vi "Gas Rack MAIN (RT).vi"() -> ()   [LabVIEW 2013]
uses:
  TypeDef/Controller Names.ctl
  TypeDef/Command Cluster.ctl
  TypeDef/DataCluster.ctl
  TCP/PC/Event Mode.ctl
  CAN Communication/CAN Mode.ctl
  TCP/RT/RTsend PCrecv CMD.ctl
  RT subVIs/Controls/Stream RT FIFO Mode.ctl
  TypeDef/TCP Cluster.ctl
  TypeDef/Stability Cluster.ctl
  <vilib>/FPGAPlugInAG/sbRIO-9626/niLvFpga_Open_sbRIO-9626.vi
  <vilib>/rvi/interface/common/dynamic/niFpgaDynamicAddResources.vi
  <vilib>/rvi/interface/common/niFpgaWaitOnOcc.vi
  <vilib>/Utility/error.llb/Error Cluster From Error Code.vi
  <vilib>/rvi/errors/niLvFpgaAdjustHostInterfaceError.vi
  <vilib>/FPGAPlugInAG/Dynamic/niLvFpga_Reset_Dynamic.vi
  <vilib>/FPGAPlugInAG/Dynamic/niLvFpga_Run_Dynamic.vi
  <vilib>/rvi/interface/nirviOpenFPGA/nirviOpenFPGA.xnode
  FPGA Bitfiles/Portable Gas Rack.lvbitx
  FPGA/Portable Gas Rack Main (FPGA).vi
  <vilib>/rvi/interface/nirviReadWriteControl/nirviReadWriteControl.xnode
  <vilib>/rvi/interface/nirviMethod/nirviMethod.xnode
  <vilib>/NI_Real-Time Target Support.lvlib
  <vilib>/rvi/interface/Simulation/niFpgaSimulationCallBeginRW.vi
  <vilib>/ptbypt/NI_PtbyPt.lvlib
  <vilib>/FPGAPlugInAG/Dynamic/niLvFpga_ReadFifo_Dynamic.vi
  <vilib>/rvi/errors/niLvFpgaMergeErrorWithErrorCode.vi
  NiFpgaLv.dll
panel:
  in  "DesiredCluster":T1
  in  "Enable Graphs":bool
  out "time 3":dbl
  out "time 2":dbl
  out "time":dbl
  out "Ave Data Cluster":T2 {"Efficiency (%)" format="%#_6f"; "Speed (RPM)" format="%#.1f"; "Fuel Temp (C)" format="%.1f"; "Controller Current (A)" format="%.2f"; "Controller Voltage (V)" format="%.2f"; "Flow (L/H)" format="%.1f"; "Pressure (kPA)" format="%.1f"; "Pump Current (Arms)" format="%.2f"; "Pump Voltage (V)" format="%#.2f"}
  in  "Tab Control Config":enum32{"PID/slew", "Cal/Hidden"}(tab)
  in  "SaveConfig":bool
  in  "ControlArray":T3(array[cluster])=[{"Name"="Volt_Direct", "PI Far->Close"=[], "FFinfo"={"FF_m"=0.0, "FF_b"=0.0}, "Limits"={"StepSize"=1e-05, "Max"=10.0, "Min"=0.0, "IndMin"=0.0}}, {"Name"="Volt_Flow", "PI Far->Close"=[], "FFinfo"={"FF_m"=0.0, "FF_b"=0.0}, "Limits"={"StepSize"=1e-05, "Max"=10.0, "Min"=0.0, "IndMin"=0.0}}, {"Name"="Volt_Speed", "PI Far->Close"=[], "FFinfo"={"FF_m"=0.0, "FF_b"=0.0}, "Limits"={"StepSize"=1e-05, "Max"=10.0, "Min"=0.0, "IndMin"=0.0}}, {"Name"="Pres_Direct", "PI Far->Close"=[], "FFinfo"={"FF_m"=0.0, "FF_b"=0.0}, "Limits"={"StepSize"=1e-05, "Max"=10.0, "Min"=0.0, "IndMin"=0.0}}, {"Name"="Pres_Flow", "PI Far->Close"=[], "FFinfo"={"FF_m"=0.0, "FF_b"=0.0}, "Limits"={"StepSize"=1e-05, "Max"=10.0, "Min"=0.0, "IndMin"=0.0}}, {"Name"="Pres_Speed", "PI Far->Close"=[], "FFinfo"={"FF_m"=0.0, "FF_b"=0.0}, "Limits"={"StepSize"=1e-05, "Max"=10.0, "Min"=0.0, "IndMin"=0.0}}, {"Name"="CMD_Direct", "PI Far->Close"=[], "FFinfo"={"FF_m"=0.0, "FF_b"=0.0}, "Limits"={"StepSize"=1e-05, "Max"=10.0, "Min"=0.0, "IndMin"=0.0}}, {"Name"="CMD_Flow", "PI Far->Close"=[], "FFinfo"={"FF_m"=0.0, "FF_b"=0.0}, "Limits"={"StepSize"=1e-05, "Max"=10.0, "Min"=0.0, "IndMin"=0.0}}, {"Name"="CMD_Speed", "PI Far->Close"=[], "FFinfo"={"FF_m"=0.0, "FF_b"=0.0}, "Limits"={"StepSize"=1e-05, "Max"=10.0, "Min"=0.0, "IndMin"=0.0}}]
  out "Speed":dbl
  in  "Max Window":dbl=1400.0 format="%.4f"
  in  "Min Window":dbl=300.0 format="%.4f"
  in  "CAN CMD":u16
  out "Speed Loop Time":dbl
  out "Actual Loop Time 2":u32
  in  "Count 2(uS)":u32=35
  out "Actual Loop Time":u32
  in  "Count 1(uS)":u32=100
  in  "Brushed Speed":bool
  in  "Stream Stop":bool
  in  "CommSegs":i32
  out "PrevCalDate":i32
  in  "CmdCluster":T1
  out "PresSig":dbl
  out "VSig":dbl
  in  "VDirect":dbl
  in  "DirectV?":bool
  in  "DirectPres?":bool
  in  "PresDirect":dbl
  in  "PS Enable":bool
  out "Controller Name":T4
  out "Total (%)":dbl
  in  "GraphTab":enum32{"Page 1", "Page 2"}(tab)=enum."Page 2"
  out "WFG1":dbl[][](graph)
  out "WFG2":dbl[][](graph)
  out "WFG3":dbl[][](graph)
  out "WFG6":dbl[][](graph)
  out "WFG5":dbl[][](graph)
  out "WFG4":dbl[][](graph)
  # "Should be 0.1"
  # "CalDate is frozen to 3/8/17"
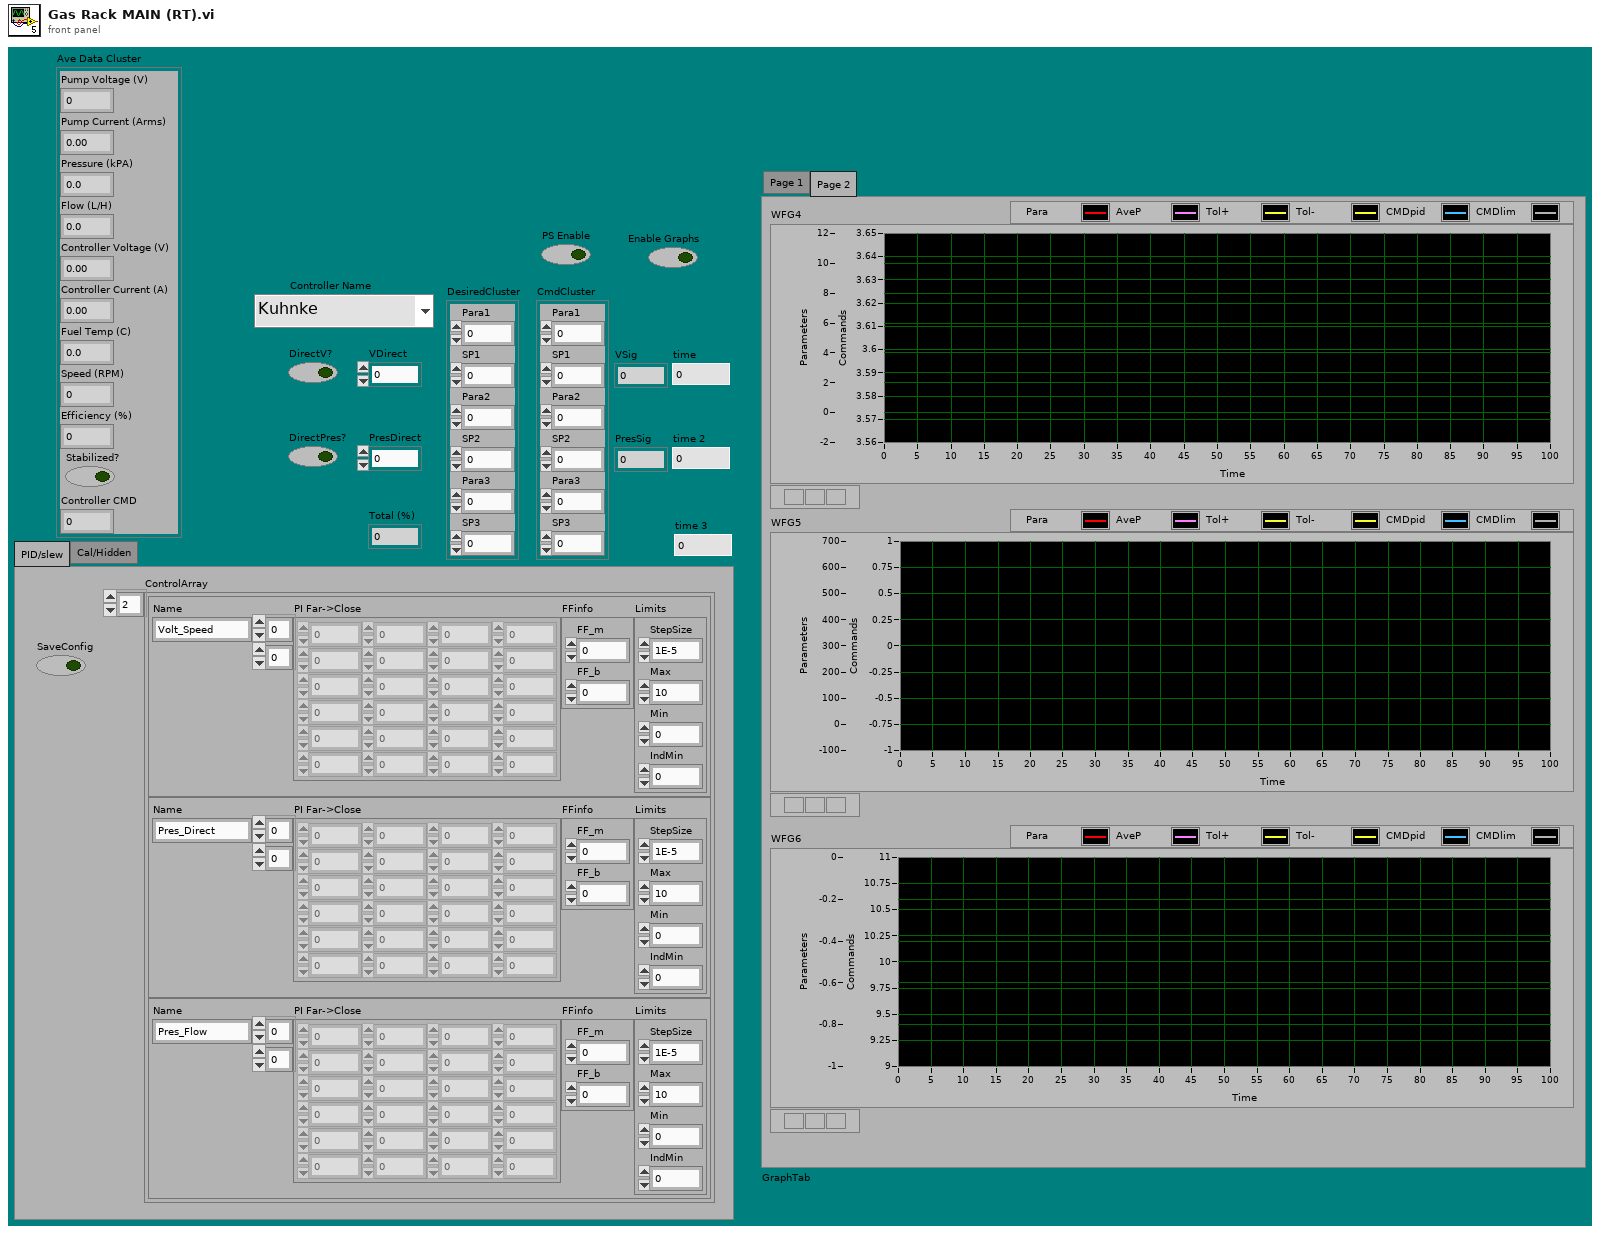
[diagram p1: front panel]
types:
  T1 = typedef "Command Cluster.ctl" = cluster{"Para1":i32, "SP1":dbl, "Para2":i32, "SP2":dbl, "Para3":i32, "SP3":dbl}
  T2 = typedef "DataCluster.ctl" = cluster{"Pump Voltage (V)":dbl, "Pump Current (Arms)":dbl, "Pressure (kPA)":dbl, "Flow (L/H)":dbl, "Controller Voltage (V)":dbl, "Controller Current (A)":dbl, "Fuel Temp (C)":dbl, "Speed (RPM)":dbl, "Efficiency (%)":dbl, "Stabilized?":bool, "Controller CMD":dbl}
  T3 = cluster{"Name":string, "PI Far->Close":dbl[][], "FFinfo":cluster{"FF_m":dbl, "FF_b":dbl}, "Limits":cluster{"StepSize":dbl, "Max":dbl, "Min":dbl, "IndMin":dbl}}[]
  T4 = typedef "Controller Names.ctl" = enum16{"Kuhnke", "McLaren", "Helbako BLDC", "Conti", "Hella E4LMF", "Hella E4LMD", "Hella E4DCG 20mm", "Hella E4DCG 30mm", "Helbako (old)", "TI PWM", "PSA", "Hella Hyundai Gas", "Hella Hyundai Diesel", "8 Comm", "10 Comm", "8 Comm Hella FCA", "10 Comm Hella FCA", "8 Comm Omron", "10 Comm Omron", "8 Comm Nissan", "10 Comm Nissan"}
  T5 = cluster{"Controller Name":T4, "CommSeg":i32, "PWM?":bool, "Frequency":i32, "Low Command":dbl, "High Command":dbl, "Stop Command":dbl, "Command Step":dbl, "Solenoid Stop?":bool, "Controller?":bool, "Name":string, "Indirect Nonzero CMD":dbl}[]
  T6 = cluster{"Controller Name":T4, "CommSeg":i32, "PWM?":bool, "Frequency":i32, "Low Command":dbl, "High Command":dbl, "Stop Command":dbl, "Command Step":dbl, "Solenoid Stop?":bool, "Controller?":bool, "Name":string, "Indirect Nonzero CMD":dbl}
  T7 = cluster{"Name":string, "PI Far->Close":cluster{"Slew":dbl, "Kp":dbl, "Ki":dbl}[], "Limits":cluster{"StepSize":dbl, "Max":dbl, "Min":dbl}, "Cutoffs":cluster{"Middle":dbl, "Close":dbl}, "FFinfo":cluster{"FF_m":dbl, "FF_b":dbl}}[]
  T8 = cluster{"Stability Reads":i32, "Stability1":i32, "Stability2":i32, "Stability3":i32}
  T9 = typedef "RTsend PCrecv CMD.ctl" = enum16{"Data", "Connected?", "CalFileDate"}
  T10 = typedef "CAN Mode.ctl" = enum16{"Init", "Read", "Write", "Close"}
  T11 = typedef "Event Mode.ctl" = enum16{"Init", "Get", "Set", "Destroy"}
  T12 = cluster{"CommandCluster":T1, "Deadhead?":bool, "FPGA Data Rate (sec)":dbl, "FPGA Data Timer":dbl, "PC Data Rate (sec)":dbl, "PC Data Timer":dbl, "InstDataCluster":T2, "Controller":cluster{"Controller Name":T4, "CommSeg":i32, "PWM?":bool, "Frequency":i32, "Low Command":dbl, "High Command":dbl, "Stop Command":dbl, "Command Step":dbl, "Solenoid Stop?":bool, "Controller?":bool, "Name":string, "Indirect Nonzero CMD":dbl}, "PWM Period (ticks)":u32, "Tolerances":dbl[], "Cal Coeffs":dbl[][], "PS Enable":bool, "StabilityCluster":cluster{"Stability Reads":i32, "Stability1":i32, "Stability2":i32, "Stability3":i32}, "AveDataCluster":T2, "CMD Scaler":dbl, "Controller List":cluster{"Controller Name":T4, "CommSeg":i32, "PWM?":bool, "Frequency":i32, "Low Command":dbl, "High Command":dbl, "Stop Command":dbl, "Command Step":dbl, "Solenoid Stop?":bool, "Controller?":bool, "Name":string, "Indirect Nonzero CMD":dbl}[], "VandPLimit":dbl[], "FreezeCmdPID":bool, "DesiredCluster":T1, "Version":u8, "ControlArray":cluster{"Name":string, "PI Far->Close":dbl[][], "FFinfo":cluster{"FF_m":dbl, "FF_b":dbl}, "Limits":cluster{"StepSize":dbl, "Max":dbl, "Min":dbl, "IndMin":dbl}}[], "TolBands":dbl[][], "NeedleValve":bool}
  T13 = typedef "TCP Cluster.ctl" = cluster{"Command":string, "FlattenedData":string}
  T14 = cluster{"CommandCluster":T1, "DesiredCluster":T1}
  T15 = typedef "Stream RT FIFO Mode.ctl" = enum16{"Create", "Write", "Read", "Delete"}
  T16 = typedef "PCsend RTrecv CMD.ctl" = enum16{"ConnSettings", "Connect", "CMD", "Controller", "PSenable", "ReqCalDate", "Tolerances", "Stable Trigger", "Stop", "VPLimits", "NeedleValve", "SpeedWindow", "FreezeCmdPID"}
  T17 = typedef "Stability Cluster.ctl" = cluster{"Voltage Tolerances":dbl, "Pressure Tolerances":dbl, "Flow Tolerances":dbl, "Speed Tolerances":dbl, "Stable Count (sec)":dbl}
  T18 = cluster{"Pump Voltage":fxp<+/-,25,15>, "Pump Current":fxp<+/-,25,15>, "Pressure":fxp<+/-,25,15>, "Flow":fxp<+/-,25,15>, "Controller Voltage":fxp<+/-,25,15>, "Controller Current":fxp<+/-,25,15>, "Temperature":fxp<+/-,25,15>, "Speed":fxp<+/-,25,15>}
  T19 = cluster{"[0]":dbl, "[1]":dbl, "[2]":dbl, "[3]":dbl, "[4]":dbl, "[5]":dbl, "[6]":dbl, "[7]":dbl}
  T20 = typedef "NI_Real-Time Target Support.lvlib/RT CPU Load.ctl" = cluster{"Total (%)":dbl, "Time Critical (%)":dbl, "Timed Structures (%)":dbl, "High (%)":dbl, "Above Normal (%)":dbl, "Normal (%)":dbl, "Background (%)":dbl, "Idle (%)":dbl, "ISR (%)":dbl}
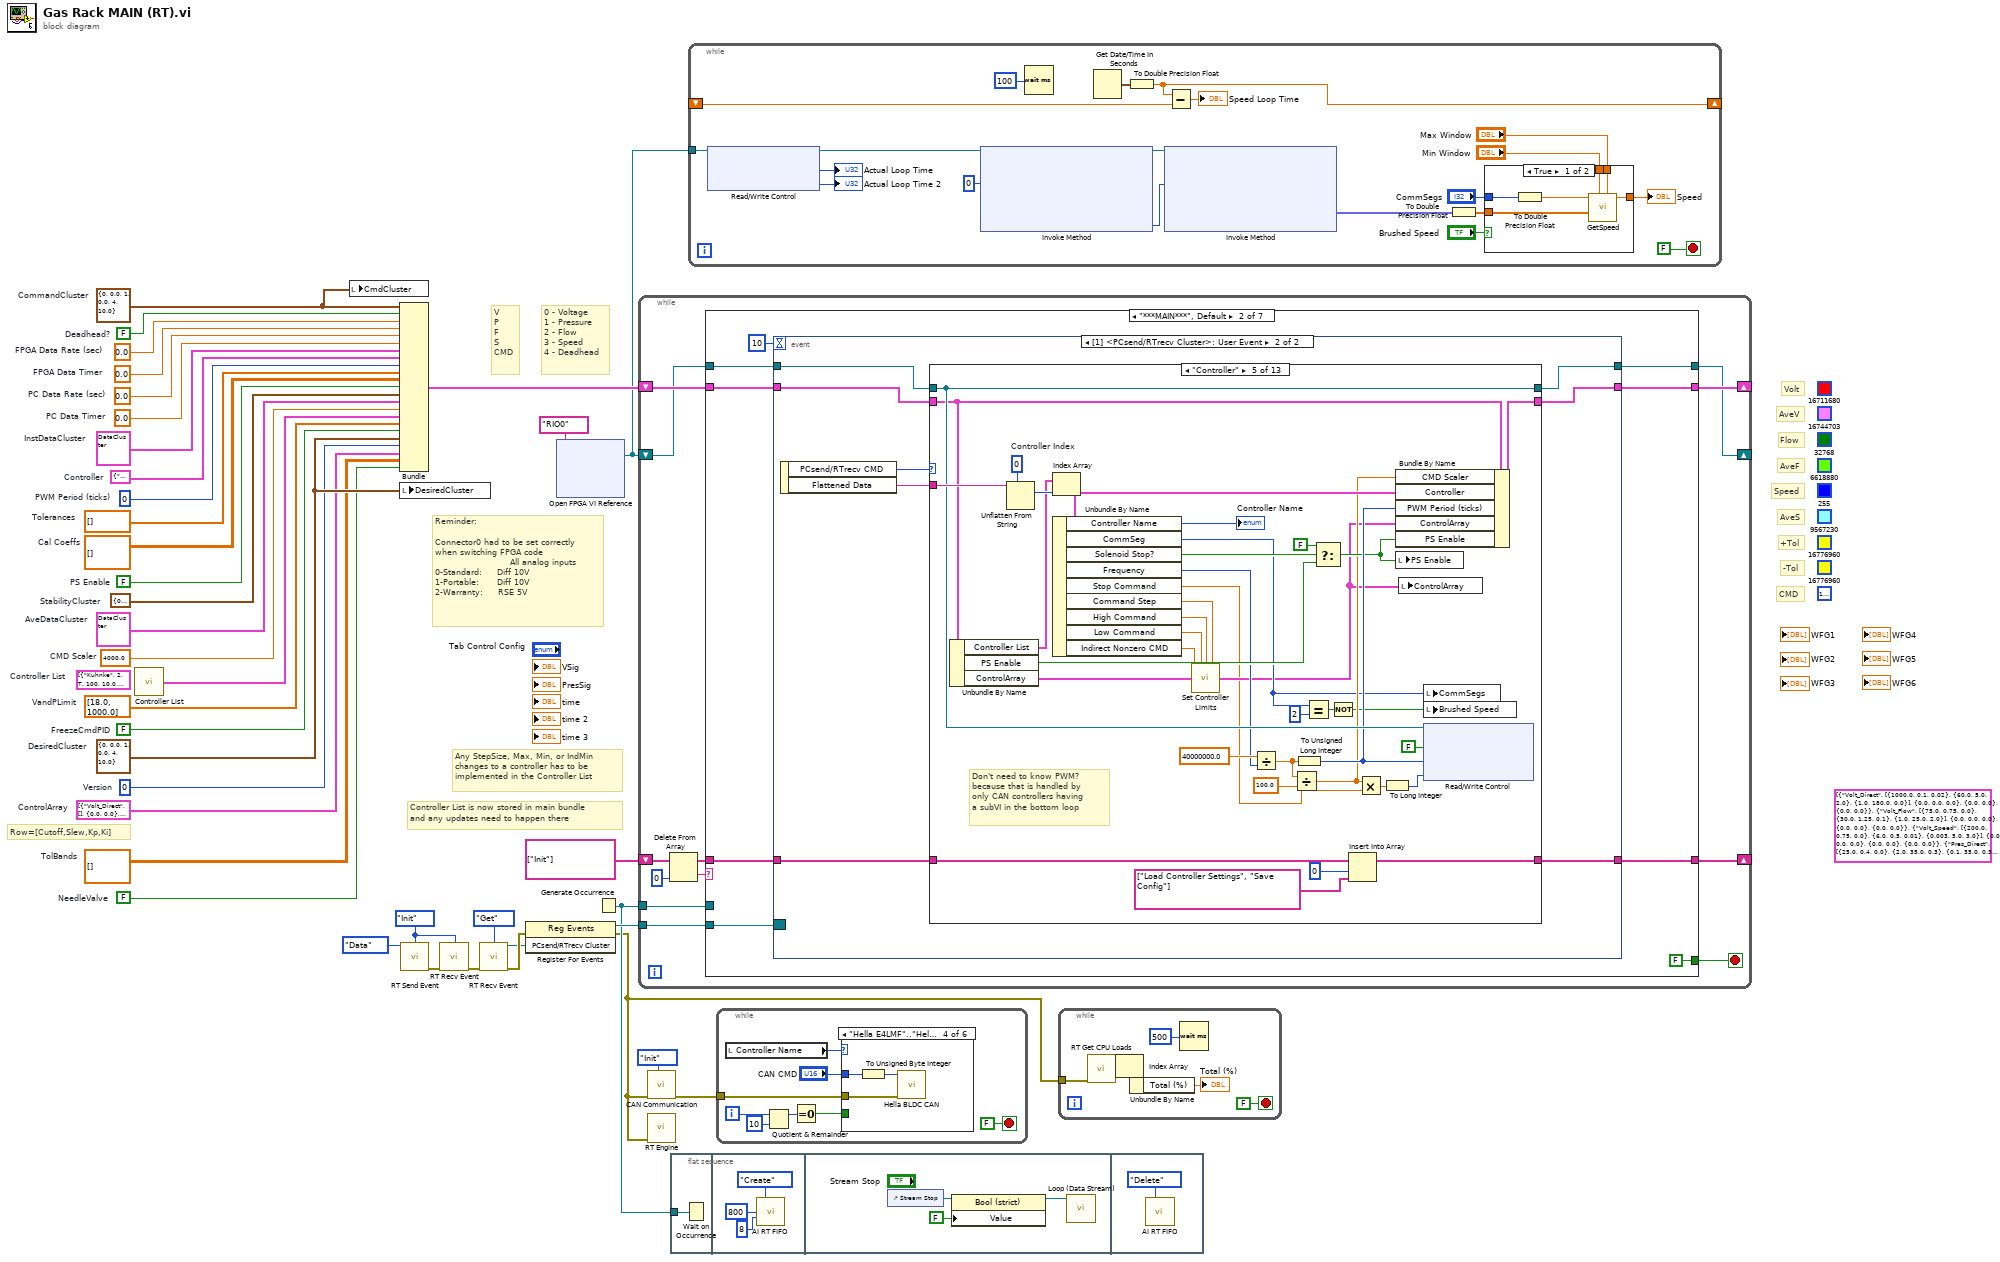
[diagram p0: block diagram]
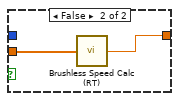
[diagram p2: hidden frame]
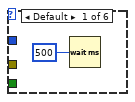
[diagram p3: hidden frame]
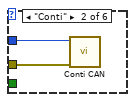
[diagram p4: hidden frame]
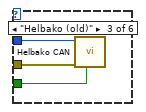
[diagram p5: hidden frame]
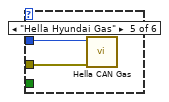
[diagram p6: hidden frame]
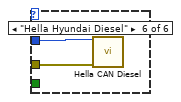
[diagram p7: hidden frame]
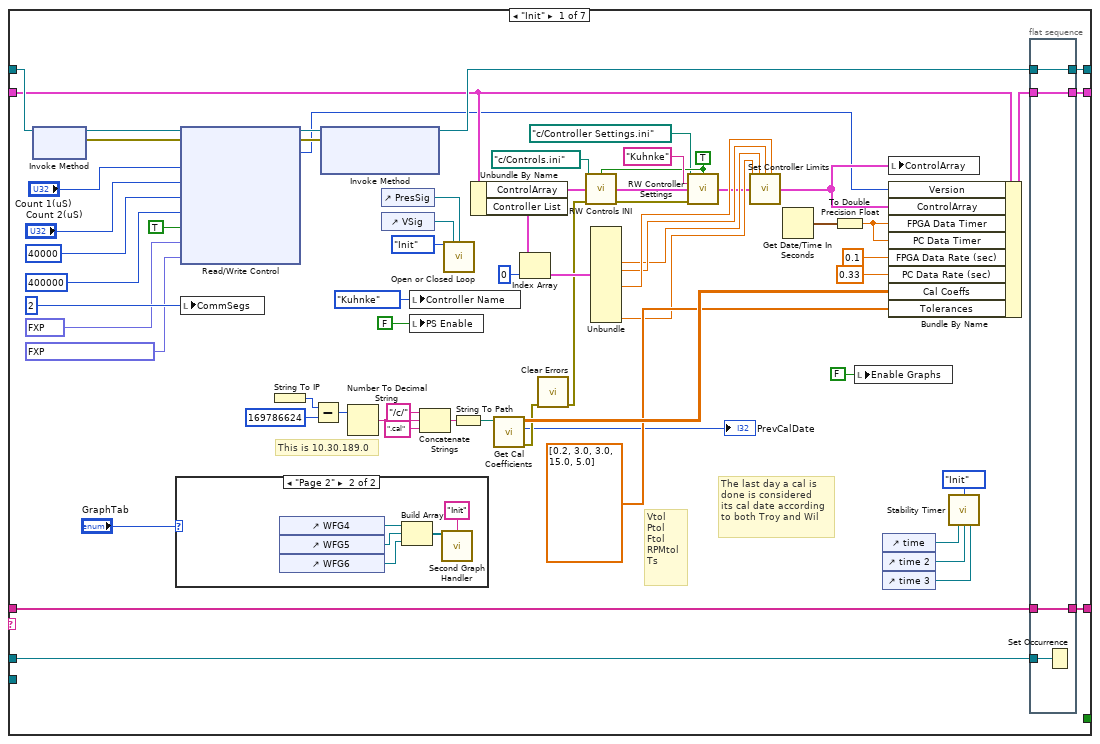
[diagram p8: hidden frame]
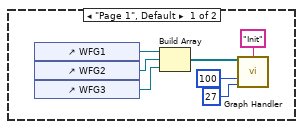
[diagram p9: hidden frame]
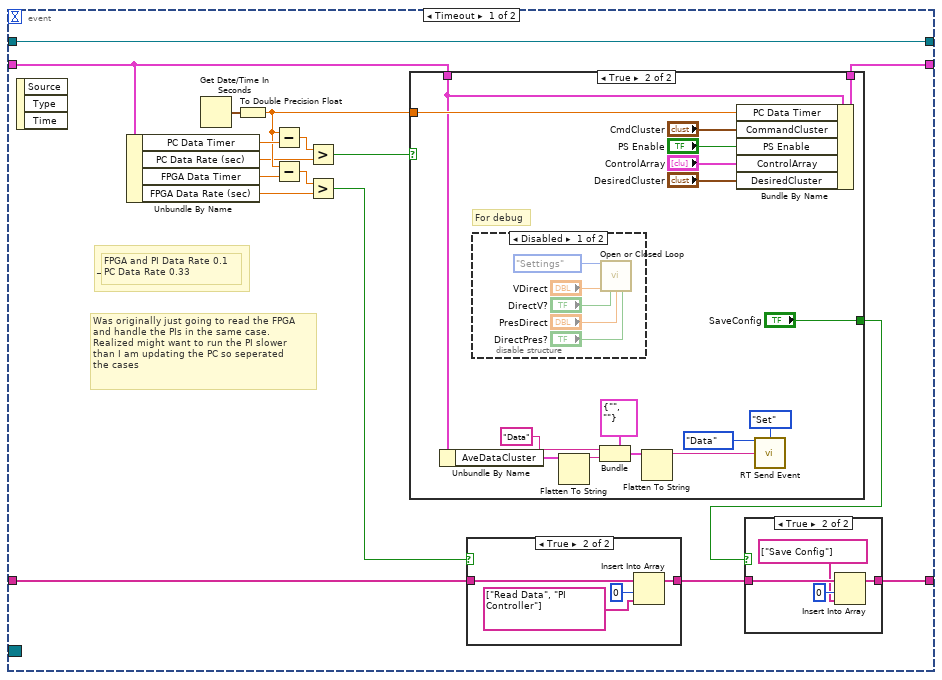
[diagram p10: hidden frame]
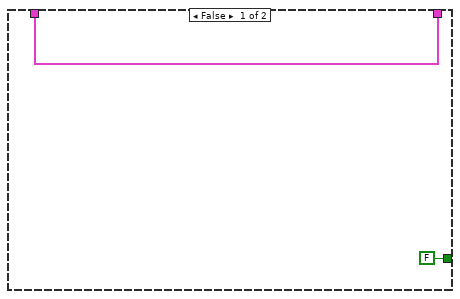
[diagram p13: hidden frame]
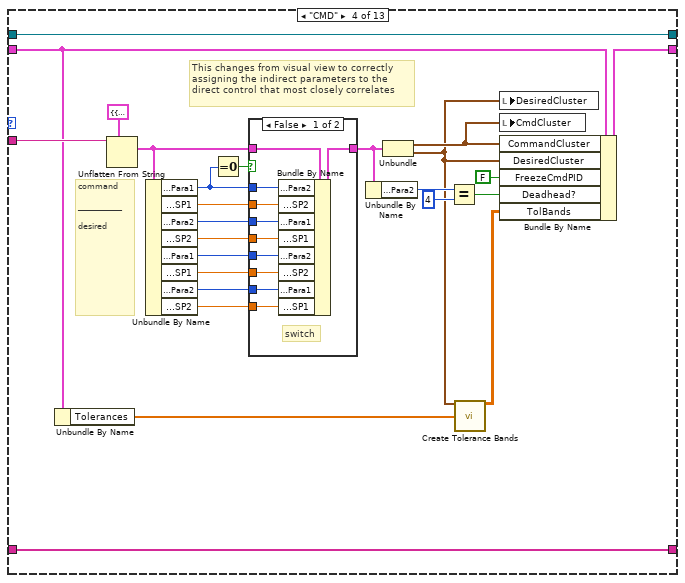
[diagram p18: hidden frame]
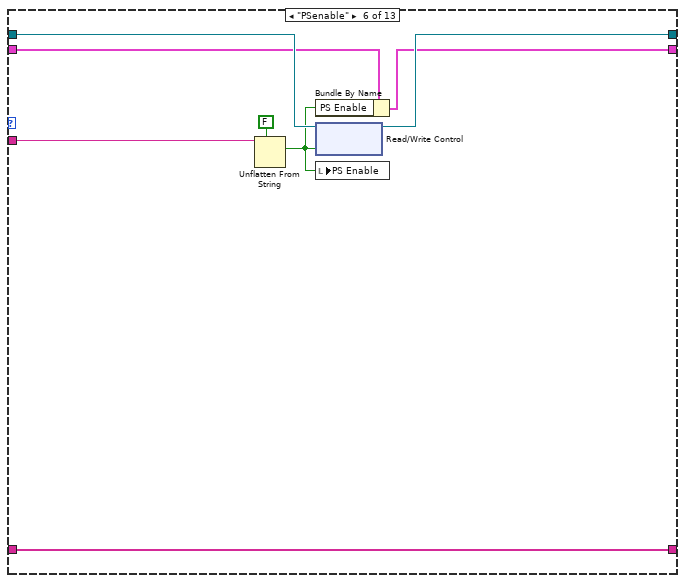
[diagram p20: hidden frame]
diagram:
  w1 = FALSE  # NeedleValve
  w2 = dbl[][] []  # TolBands
  w3 = u8 0  # Version
  w4 = T3 [{"Name"="Volt_Direct", "PI Far->Close"=[], "FFinfo"={"FF_m"=0.0, "FF_b"=0.0}, "Limits"={"StepSize"=1e-05, "Max"=10.0, "Min"=0.0, "IndMin"=0.0}}, {"Name"="Volt_Flow", "PI Far->Close"=[], "FFinfo"={"FF_m"=0.0, "FF_b"=0.0}, "Limits"={"StepSize"=1e-05, "Max"=10.0, "Min"=0.0, "IndMin"=0.0}}, {"Name"="Volt_Speed", "PI Far->Close"=[], "FFinfo"={"FF_m"=0.0, "FF_b"=0.0}, "Limits"={"StepSize"=1e-05, "Max"=10.0, "Min"=0.0, "IndMin"=0.0}}, {"Name"="Pres_Direct", "PI Far->Close"=[], "FFinfo"={"FF_m"=0.0, "FF_b"=0.0}, "Limits"={"StepSize"=1e-05, "Max"=10.0, "Min"=0.0, "IndMin"=0.0}}, {"Name"="Pres_Flow", "PI Far->Close"=[], "FFinfo"={"FF_m"=0.0, "FF_b"=0.0}, "Limits"={"StepSize"=1e-05, "Max"=10.0, "Min"=0.0, "IndMin"=0.0}}, {"Name"="Pres_Speed", "PI Far->Close"=[], "FFinfo"={"FF_m"=0.0, "FF_b"=0.0}, "Limits"={"StepSize"=1e-05, "Max"=10.0, "Min"=0.0, "IndMin"=0.0}}, {"Name"="CMD_Direct", "PI Far->Close"=[], "FFinfo"={"FF_m"=0.0, "FF_b"=0.0}, "Limits"={"StepSize"=1e-05, "Max"=10.0, "Min"=0.0, "IndMin"=0.0}}, {"Name"="CMD_Flow", "PI Far->Close"=[], "FFinfo"={"FF_m"=0.0, "FF_b"=0.0}, "Limits"={"StepSize"=1e-05, "Max"=10.0, "Min"=0.0, "IndMin"=0.0}}, {"Name"="CMD_Speed", "PI Far->Close"=[], "FFinfo"={"FF_m"=0.0, "FF_b"=0.0}, "Limits"={"StepSize"=1e-05, "Max"=10.0, "Min"=0.0, "IndMin"=0.0}}]  # ControlArray
  w5 = T1 {"Para1"=0, "SP1"=0.0, "Para2"=1, "SP2"=0.0, "Para3"=4, "SP3"=10.0}  # DesiredCluster
  w6 = FALSE  # FreezeCmdPID
  (unwired) T5 [{"Controller Name"=enum."Kuhnke", "CommSeg"=2, "PWM?"=TRUE, "Frequency"=100, "Low Command"=10.0, "High Command"=90.0, "Stop Command"=10.0, "Command Step"=0.1, "Solenoid Stop?"=FALSE, "Controller?"=TRUE, "Name"="Kuhnke", "Indirect Nonzero CMD"=15.0}, {"Controller Name"=enum."Helbako BLDC", "CommSeg"=2, "PWM?"=TRUE, "Frequency"=100, "Low Command"=10.0, "High Command"=90.0, "Stop Command"=10.0, "Command Step"=0.1, "Solenoid Stop?"=FALSE, "Controller?"=TRUE, "Name"="Helbako BLDC", "Indirect Nonzero CMD"=15.0}, {"Controller Name"=enum."Conti", "CommSeg"=2, "PWM?"=FALSE, "Frequency"=100, "Low Command"=0.0, "High Command"=800.0, "Stop Command"=0.0, "Command Step"=1.0, "Solenoid Stop?"=FALSE, "Controller?"=TRUE, "Name"="Conti", "Indirect Nonzero CMD"=0.0}, {"Controller Name"=enum."Hella E4LMF", "CommSeg"=2, "PWM?"=FALSE, "Frequency"=100, "Low Command"=0.0, "High Command"=100.0, "Stop Command"=0.0, "Command Step"=1.0, "Solenoid Stop?"=FALSE, "Controller?"=TRUE, "Name"="Hella BLDC Screw", "Indirect Nonzero CMD"=10.0}, {"Controller Name"=enum."Helbako (old)", "CommSeg"=2, "PWM?"=FALSE, "Frequency"=100, "Low Command"=0.0, "High Command"=100.0, "Stop Command"=0.0, "Command Step"=1.0, "Solenoid Stop?"=FALSE, "Controller?"=TRUE, "Name"="Hella BLDC Turbine", "Indirect Nonzero CMD"=10.0}, {"Controller Name"=enum."Helbako (old)", "CommSeg"=2, "PWM?"=FALSE, "Frequency"=100, "Low Command"=0.0, "High Command"=100.0, "Stop Command"=0.0, "Command Step"=0.1, "Solenoid Stop?"=FALSE, "Controller?"=TRUE, "Name"="Helbako (old)", "Indirect Nonzero CMD"=0.0}, {"Controller Name"=enum."TI PWM", "CommSeg"=2, "PWM?"=TRUE, "Frequency"=100, "Low Command"=0.0, "High Command"=100.0, "Stop Command"=0.0, "Command Step"=0.1, "Solenoid Stop?"=FALSE, "Controller?"=TRUE, "Name"="TI PWM", "Indirect Nonzero CMD"=0.0}, {"Controller Name"=enum."PSA", "CommSeg"=2, "PWM?"=TRUE, "Frequency"=100, "Low Command"=5.0, "High Command"=95.0, "Stop Command"=5.0, "Command Step"=0.1, "Solenoid Stop?"=FALSE, "Controller?"=TRUE, "Name"="PSA", "Indirect Nonzero CMD"=5.0}, {"Controller Name"=enum."Hella Hyundai Diesel", "CommSeg"=2, "PWM?"=FALSE, "Frequency"=100, "Low Command"=0.0, "High Command"=800.0, "Stop Command"=0.0, "Command Step"=1.0, "Solenoid Stop?"=TRUE, "Controller?"=TRUE, "Name"="Hella Gas", "Indirect Nonzero CMD"=0.0}, {"Controller Name"=enum."8 Comm", "CommSeg"=10, "PWM?"=FALSE, "Frequency"=100, "Low Command"=370.0, "High Command"=461.0, "Stop Command"=370.0, "Command Step"=1.0, "Solenoid Stop?"=TRUE, "Controller?"=TRUE, "Name"="Hella Diesel", "Indirect Nonzero CMD"=370.0}, {"Controller Name"=enum."8 Comm", "CommSeg"=8, "PWM?"=FALSE, "Frequency"=150, "Low Command"=0.0, "High Command"=1.0, "Stop Command"=0.0, "Command Step"=1.0, "Solenoid Stop?"=FALSE, "Controller?"=FALSE, "Name"="8 Comm", "Indirect Nonzero CMD"=0.0}, {"Controller Name"=enum."10 Comm", "CommSeg"=10, "PWM?"=FALSE, "Frequency"=150, "Low Command"=0.0, "High Command"=1.0, "Stop Command"=0.0, "Command Step"=1.0, "Solenoid Stop?"=FALSE, "Controller?"=FALSE, "Name"="10 Comm", "Indirect Nonzero CMD"=0.0}, {"Controller Name"=enum."10 Comm Hella FCA", "CommSeg"=8, "PWM?"=TRUE, "Frequency"=150, "Low Command"=0.0, "High Command"=50.0, "Stop Command"=80.0, "Command Step"=0.1, "Solenoid Stop?"=FALSE, "Controller?"=TRUE, "Name"="8 Comm Hella", "Indirect Nonzero CMD"=0.0}, {"Controller Name"=enum."8 Comm Omron", "CommSeg"=10, "PWM?"=TRUE, "Frequency"=150, "Low Command"=0.0, "High Command"=50.0, "Stop Command"=80.0, "Command Step"=0.1, "Solenoid Stop?"=FALSE, "Controller?"=TRUE, "Name"="10 Comm Hella", "Indirect Nonzero CMD"=0.0}, {"Controller Name"=enum."8 Comm Omron", "CommSeg"=8, "PWM?"=TRUE, "Frequency"=150, "Low Command"=5.0, "High Command"=50.0, "Stop Command"=75.0, "Command Step"=0.1, "Solenoid Stop?"=FALSE, "Controller?"=TRUE, "Name"="8 Comm Omron", "Indirect Nonzero CMD"=5.0}, {"Controller Name"=enum."10 Comm Omron", "CommSeg"=10, "PWM?"=TRUE, "Frequency"=150, "Low Command"=5.0, "High Command"=50.0, "Stop Command"=75.0, "Command Step"=0.1, "Solenoid Stop?"=FALSE, "Controller?"=TRUE, "Name"="10 Comm Omron", "Indirect Nonzero CMD"=5.0}, {"Controller Name"=enum."8 Comm Nissan", "CommSeg"=8, "PWM?"=TRUE, "Frequency"=10, "Low Command"=50.0, "High Command"=90.0, "Stop Command"=50.0, "Command Step"=0.1, "Solenoid Stop?"=TRUE, "Controller?"=TRUE, "Name"="8 Comm Nissan", "Indirect Nonzero CMD"=50.0}, {"Controller Name"=enum."10 Comm Nissan", "CommSeg"=10, "PWM?"=TRUE, "Frequency"=10, "Low Command"=50.0, "High Command"=90.0, "Stop Command"=50.0, "Command Step"=0.1, "Solenoid Stop?"=TRUE, "Controller?"=TRUE, "Name"="10 Comm Nissan", "Indirect Nonzero CMD"=50.0}]  # Controller List
  w11 = T6 {"Controller Name"=enum."Kuhnke", "CommSeg"=2, "PWM?"=TRUE, "Frequency"=100, "Low Command"=10.0, "High Command"=100.0, "Stop Command"=10.0, "Command Step"=0.1, "Solenoid Stop?"=FALSE, "Controller?"=TRUE, "Name"="Kuhnke", "Indirect Nonzero CMD"=15.0}  # Controller
  w12 = dbl[] [18.0, 1000.0]  # VandPLimit
  (unwired) T7 [{"Name"="Volt_Direct", "PI Far->Close"=[{"Slew"=1000.0, "Kp"=0.1, "Ki"=0.02}, {"Slew"=60.0, "Kp"=5.0, "Ki"=2.0}, {"Slew"=1.0, "Kp"=180.0, "Ki"=0.0}], "Limits"={"StepSize"=0.0, "Max"=0.0, "Min"=0.0}, "Cutoffs"={"Middle"=0.0, "Close"=0.0}, "FFinfo"={"FF_m"=0.0, "FF_b"=0.0}}, {"Name"="Volt_Flow", "PI Far->Close"=[{"Slew"=75.0, "Kp"=0.75, "Ki"=0.0}, {"Slew"=30.0, "Kp"=1.25, "Ki"=0.1}, {"Slew"=1.0, "Kp"=25.0, "Ki"=2.0}], "Limits"={"StepSize"=0.0, "Max"=0.0, "Min"=0.0}, "Cutoffs"={"Middle"=0.0, "Close"=0.0}, "FFinfo"={"FF_m"=0.0, "FF_b"=0.0}}, {"Name"="Volt_Speed", "PI Far->Close"=[{"Slew"=200.0, "Kp"=0.75, "Ki"=0.0}, {"Slew"=6.0, "Kp"=0.5, "Ki"=0.01}, {"Slew"=0.003, "Kp"=5.0, "Ki"=3.0}], "Limits"={"StepSize"=0.0, "Max"=0.0, "Min"=0.0}, "Cutoffs"={"Middle"=0.0, "Close"=0.0}, "FFinfo"={"FF_m"=0.0, "FF_b"=0.0}}, {"Name"="Pres_Direct", "PI Far->Close"=[{"Slew"=25.0, "Kp"=0.4, "Ki"=0.0}, {"Slew"=2.0, "Kp"=35.0, "Ki"=0.3}, {"Slew"=0.1, "Kp"=35.0, "Ki"=0.3}], "Limits"={"StepSize"=0.0, "Max"=0.0, "Min"=0.0}, "Cutoffs"={"Middle"=0.0, "Close"=0.0}, "FFinfo"={"FF_m"=0.0, "FF_b"=0.0}}, {"Name"="Pres_Flow", "PI Far->Close"=[{"Slew"=65.0, "Kp"=-5.0, "Ki"=0.0}, {"Slew"=25.0, "Kp"=-25.0, "Ki"=-1.0}, {"Slew"=0.0, "Kp"=-250.0, "Ki"=-120.0}], "Limits"={"StepSize"=0.0, "Max"=0.0, "Min"=0.0}, "Cutoffs"={"Middle"=0.0, "Close"=0.0}, "FFinfo"={"FF_m"=0.0, "FF_b"=0.0}}, {"Name"="Pres_Speed", "PI Far->Close"=[{"Slew"=50.0, "Kp"=-100.0, "Ki"=-10.0}, {"Slew"=1.0, "Kp"=-50.0, "Ki"=-7.5}, {"Slew"=1.0, "Kp"=-50.0, "Ki"=-7.5}], "Limits"={"StepSize"=0.0, "Max"=0.0, "Min"=0.0}, "Cutoffs"={"Middle"=0.0, "Close"=0.0}, "FFinfo"={"FF_m"=0.0, "FF_b"=0.0}}, {"Name"="CMD_Direct", "PI Far->Close"=[{"Slew"=1.0, "Kp"=1.0, "Ki"=0.1}, {"Slew"=1.0, "Kp"=1.0, "Ki"=0.1}, {"Slew"=1.0, "Kp"=1.0, "Ki"=0.1}], "Limits"={"StepSize"=0.0, "Max"=0.0, "Min"=0.0}, "Cutoffs"={"Middle"=0.0, "Close"=0.0}, "FFinfo"={"FF_m"=0.0, "FF_b"=0.0}}, {"Name"="CMD_Flow", "PI Far->Close"=[{"Slew"=650.0, "Kp"=10.0, "Ki"=1.0}, {"Slew"=50.0, "Kp"=100.0, "Ki"=2.0}, {"Slew"=10.0, "Kp"=140.0, "Ki"=5.0}], "Limits"={"StepSize"=0.0, "Max"=0.0, "Min"=0.0}, "Cutoffs"={"Middle"=0.0, "Close"=0.0}, "FFinfo"={"FF_m"=0.0, "FF_b"=0.0}}, {"Name"="CMD_Speed", "PI Far->Close"=[{"Slew"=999999.0, "Kp"=0.0, "Ki"=0.0}, {"Slew"=999999.0, "Kp"=0.0, "Ki"=0.0}, {"Slew"=999999.0, "Kp"=0.0, "Ki"=0.15}], "Limits"={"StepSize"=0.0, "Max"=0.0, "Min"=0.0}, "Cutoffs"={"Middle"=0.0, "Close"=0.0}, "FFinfo"={"FF_m"=0.0, "FF_b"=0.0}}] ("ControlArray")
  (unwired) u32 16744703
  (unwired) u32 6618880
  (unwired) u32 9567230
  (unwired) u32 16777226
  (unwired) u32 16776960
  (unwired) u32 16776960
  (unwired) u32 255
  (unwired) u32 32768
  (unwired) u32 16711680
  w15 = T1 {"Para1"=0, "SP1"=0.0, "Para2"=1, "SP2"=0.0, "Para3"=4, "SP3"=10.0}  # CommandCluster
  w30 = T2 {"Pump Voltage (V)"=0.0, "Pump Current (Arms)"=0.0, "Pressure (kPA)"=0.0, "Flow (L/H)"=0.0, "Controller Voltage (V)"=0.0, "Controller Current (A)"=0.0, "Fuel Temp (C)"=0.0, "Speed (RPM)"=0.0, "Efficiency (%)"=0.0, "Stabilized?"=FALSE, "Controller CMD"=0.0}  # InstDataCluster
  w13 = 4000.0  # CMD Scaler
  w14 = T2 {"Pump Voltage (V)"=0.0, "Pump Current (Arms)"=0.0, "Pressure (kPA)"=0.0, "Flow (L/H)"=0.0, "Controller Voltage (V)"=0.0, "Controller Current (A)"=0.0, "Fuel Temp (C)"=0.0, "Speed (RPM)"=0.0, "Efficiency (%)"=0.0, "Stabilized?"=FALSE, "Controller CMD"=0.0}  # AveDataCluster
  w16 = T8 {"Stability Reads"=0, "Stability1"=0, "Stability2"=0, "Stability3"=0}  # StabilityCluster
  w17 = FALSE  # PS Enable
  w18 = dbl[][] []  # Cal Coeffs
  w20 = 0.0  # PC Data Timer
  w21 = 0.0  # PC Data Rate (sec)
  w25 = FALSE  # Deadhead?
  w26 = dbl[] []  # Tolerances
  w27 = Event_Mode."Init" ("Mode")
  w29 = u32 0  # PWM Period (ticks)
  w36 = 0.0  # FPGA Data Timer
  w37 = 0.0  # FPGA Data Rate (sec)
  # "Row=[Cutoff,Slew,Kp,Ki]"
  # "Any StepSize, Max, Min, or IndMin\nchanges to a controller has to be\nimplemented in the Controller List"
  # "Controller List is now stored in main bundle\nand any updates need to happen there"
  # "CMD"
  # "-Tol"
  # "+Tol"
  # "AveS"
  # "Speed"
  # "AveF"
  # "Flow"
  # "AveV"
  # "Volt"
  # "V\nP\nF\nS\nCMD"
  # "0 - Voltage\n1 - Pressure\n2 - Flow\n3 - Speed\n4 - Deadhead"
  # "Reminder:\n\nConnector0 had to be set correctly\nwhen switching FPGA code\n                         All analog inputs\n0-Standard:     Diff 10V\n1-Portable:      Diff 10V\n2-Warranty:     RSE 5V"
  n1 = call "Controller List.vi"() -> ("Controller List"=w10:T5)  [unwired: 5 in]
  n2 = local write "CmdCluster"(w15) -> ()
  n3 = Bundle("CommandCluster"=w15, "Deadhead?"=w25, "FPGA Data Rate (sec)"=w37, "FPGA Data Timer"=w36, "PC Data Rate (sec)"=w21, "PC Data Timer"=w20, "InstDataCluster"=w30, "Controller"=w11, "PWM Period (ticks)"=w29, "Tolerances"=w26, "Cal Coeffs"=w18, "PS Enable"=w17, "StabilityCluster"=w16, "AveDataCluster"=w14, "CMD Scaler"=w13, "Controller List"=w10, "VandPLimit"=w12, "FreezeCmdPID"=w6, "DesiredCluster"=w5, "Version"=w3, "ControlArray"=w4, "TolBands"=w2, "NeedleValve"=w1) -> (w38:T12)  [unwired: 1 in]
  n4 = local write "DesiredCluster"(w5) -> ()
  n5 = call "RT Send Event.vi"("RTsend/PCrecv CMD"=RTsend_PCrecv_CMD."Data", "Mode"=w27) -> ("Error Out"=w35:errorcluster)  [unwired: 12 in, 1 out]
  n6 = call "RT Recv Event.vi"("Mode"=w27, "Error In"=w35) -> ("Error Out"=w34:errorcluster)  [unwired: 12 in, 1 out]
  n7 = call "RT Recv Event.vi"("Mode"=Event_Mode."Get", "Error In"=w34) -> ("PCsend/RTrecv Cluster"=w32:refnum<user-event>, "Error Out"=w33:errorcluster)  [unwired: 12 in]
  n8 = register-events(error in=w33, w32) -> (reference out=w31:refnum<event-registration>, error out=w7:errorcluster)  [unwired: 1 in]
  n9 = xnode ("Open FPGA VI Reference")("resource name"=tag "RIO0") -> ("FPGA VI Reference Out"=w9:refnum<k20>)  [unwired: 1 in, 1 out]
  n10 = Generate Occurrence() -> (w19:refnum<k4>)
  n11 = while {
    shift-right: [w47] -> _
    shift-left: string[] ["Init"] -> [w51]
    shift-right: [w44] -> _
    shift-left: w38 -> [w46]
    shift-right: [w42] -> _
    shift-left: w9 -> [w43]
    tunnel: w31 -> [w41]
    tunnel: w19 -> [w40]
    stop <- w45 stop-if-true
    n12 = Delete From Array(array=w51, index=0) -> (deleted portion=w48:string, array with subset deleted=w49:string[])  [unwired: 1 in]
    n13 = case shown="\"***MAIN***\", Default" w48 {
      tunnel: w49 -> [w102 w142 w360 w427 w461 w474 w487]
      tunnel: [w101 w138 w360 w426 w461 w474 w487] -> w47
      tunnel: w46 -> [w96 w141 w356 w429 w458 w467 w479]
      tunnel: [_ FALSE _ _ _ _ _] -> w45
      tunnel: [w103 w139 w358 w425 w458 w473 w486] -> w44
      tunnel: w43 -> [w116 w136 w359 w428 w460 w475 w488]
      tunnel: [w104 w135 w359 w428 w459 w475 w488] -> w42
      tunnel: w41 -> [_ w134 _ _ _ _ _]
      tunnel: w40 -> [w100 _ _ _ _ _ _]
      frame "Init" {
        w73 = TRUE ("Read (F)")
        # "The last day a cal is\ndone is considered\nits cal date according\nto both Troy and Wil"
        # "Vtol\nPtol\nFtol\nRPMtol\nTs"
        # "This is 10.30.189.0"
        n14 = xnode "Invoke Method"("FPGA VI Reference In"=w116) -> ("FPGA VI Reference Out"=w94:refnum<k20>, "error out"=w93:errorcluster)  [unwired: 1 in]
        n15 = case shown="\"Page 2\"" "GraphTab" {
          frame "Page 1", Default {
            n16 = control-ref of="WFG1"() -> (w121:refnum<vi>)
            n17 = control-ref of="WFG2"() -> (w122:refnum<vi>)
            n18 = control-ref of="WFG3"() -> (w124:refnum<vi>)
            n19 = Build Array(w121, w122, w124) -> (w123:refnum<vi>[])
            n20 = call "Graph Handler.vi"("WF Ref Array"=w123, "State"="Init", "ChSize"=100, "NumCh"=27) -> ()  [unwired: 12 in]
          }
          frame "Page 2" {
            n21 = control-ref of="WFG4"() -> (w129:refnum<vi>)
            n22 = control-ref of="WFG5"() -> (w128:refnum<vi>)
            n23 = control-ref of="WFG6"() -> (w127:refnum<vi>)
            n24 = Build Array(w129, w128, w127) -> (w126:refnum<vi>[])
            n25 = call "Second Graph Handler.vi"("WF Ref Array"=w126, "State"="Init") -> ()  [unwired: 14 in]
          }
        }
        n26 = xnode "Read/Write Control"("FPGA VI Reference In"=w94, "error in"=w93, "Count 1(uS)"="Count 1(uS)", "Count 2(uS)"="Count 2(uS)", "PWM Duty"=40000, "PWM Period (ticks)"=u32 400000, "NeedleValve"=TRUE, "Hysteresis"=fxp<+,24,5> 0.0625, "CtCuttoff"=fxp<+,24,5> 2.5416698455810547) -> ("FPGA VI Reference Out"=w91:refnum<k20>, "error out"=w92:errorcluster, "Version"=w53:u8)
        n27 = local write "CommSegs"(2 ("CommSegs")) -> ()
        n28 = String To IP() -> (0:w113:u32)  [unwired: 1 in]
        n29 = Subtract(x=w113, y=u32 169786624) -> (x-y=w112:u32)
        n30 = xnode "Invoke Method"("FPGA VI Reference In"=w91, "error in"=w92) -> ("FPGA VI Reference Out"=w106:refnum<k20>)  [unwired: 1 in, 1 out]
        n31 = Number To Decimal String(number=w112) -> (decimal integer string=w111:string)  [unwired: 1 in]
        n32 = control-ref of="PresSig"() -> (w70:refnum<vi>)
        n33 = control-ref of="VSig"() -> (w69:refnum<vi>)
        n34 = local write "Controller Name"(Controller_Names."Kuhnke" ("Controller Name")) -> ()
        n35 = local write "PS Enable"(FALSE ("PS Enable")) -> ()
        n36 = Concatenate Strings("/c/" ("string"), w111, ".cal" ("string")) -> (w108:string)
        n37 = call "Open or Closed Loop.vi"("Mode"=enum16{"Init", "Settings", "Run"}."Init", "VSig"=w69, "PresSig"=w70) -> ()  [unwired: 11 in, 2 out]
        n38 = String To Path(string=w108) -> (path=w107:path)
        n39 = Unbundle By Name(w96) -> ("ControlArray"=w62:T3, "Controller List"=w82:T5)
        n40 = call "Get Cal Coefficients.vi"("Path"=w107) -> ("Error Out"=w98:errorcluster, "PrevCalDate"=→"PrevCalDate":i32, "Cal Coefficients"=w99:dbl[][])  [unwired: 8 in]
        n41 = Index Array(array=w82, index=0) -> (element=w80:T6)
        n42 = call <vilib>:"Clear Errors.vi"("error in (no error)"=w98) -> ("error out"=w74:errorcluster)  [unwired: 6 in]
        n43 = call "RW Controls INI.vi"("Filepath"=path "c:/Controls.ini", "Read (F)"=w73, "ControlArray In"=w62, "Error In"=w74) -> ("ControlArray Out"=w61:T3, "Error Out"=w75:errorcluster)  [unwired: 10 in]
        n44 = Unbundle(w80) -> ("Low Command"=w76:dbl, "High Command"=w77:dbl, "Command Step"=w78:dbl, "Indirect Nonzero CMD"=w79:dbl)  [unwired: 8 out]
        n45 = call "RW Controller Settings.vi"("Filepath"=path "c:/Controller Settings.ini", "Read (F)"=w73, "Controller Name"="Kuhnke", "ControlArray In"=w61, "Error In"=w75) -> ("ControlArray Out"=w60:T3)  [unwired: 9 in, 1 out]
        n46 = call "Set Controller Limits.vi"("IndMin"=w79, "Min"=w76, "Max"=w77, "StepSize"=w78, "ControlArray In"=w60) -> ("ControlArray Out"=w59:T3)  [unwired: 10 in]
        n47 = Get Date/Time In Seconds() -> (seconds since 1Jan1904=w117:timestamp)
        n48 = To Double Precision Float(number=w117) -> (double precision float=w97:dbl)
        n49 = local write "Enable Graphs"(FALSE ("Enable Graphs")) -> ()
        n50 = control-ref of="time"() -> (w66:refnum<vi>)
        n51 = control-ref of="time 2"() -> (w65:refnum<vi>)
        n52 = control-ref of="time 3"() -> (w64:refnum<vi>)
        n53 = local write "ControlArray"(w59) -> ()
        n54 = Bundle By Name(cluster=w96, "Version"=w53, "ControlArray"=w59, "FPGA Data Timer"=w97, "PC Data Timer"=w97, "FPGA Data Rate (sec)"=0.1 ("PI Timer"), "PC Data Rate (sec)"=0.33 ("PC Data Timer"), "Cal Coeffs"=w99, "Tolerances"=dbl[] [0.2, 3.0, 3.0, 15.0, 5.0]) -> (w105:T12)
        n55 = call "Stability Timer.vi"("Mode"=enum16{"Init", "Run"}."Init", "time"=w66, "time 2"=w65, "time 3"=w64) -> ()  [unwired: 10 in, 2 out]
        n56 = flat-sequence {
          tunnel: w106 -> [w133]
          tunnel: w105 -> [w132]
          tunnel: [w133] -> w104
          tunnel: [w132] -> w103
          tunnel: w102 -> [w131]
          tunnel: [w131] -> w101
          tunnel: w100 -> [w130]
          frame #0 {
            n57 = Set Occurrence(w130) -> ()
          }
        }
      }
      frame "***MAIN***", Default {
        n58 = event shown="[1] <PCsend/RTrecv Cluster>: User Event" {
          selector: w134 -> [_ _]
          dyn-events: _ -> [_ _]
          timeout: 10 -> [_ _]
          tunnel: w142 -> [w143 w197]
          tunnel: w141 -> [w151 w200]
          tunnel: [w149 w199] -> w139
          tunnel: [w146 w196] -> w138
          tunnel: w136 -> [w159 w193]
          tunnel: [w159 w195] -> w135
          event Timeout {
            # "Was originally just going to read the FPGA\nand handle the PIs in the same case.\nRealized might want to run the PI slower\nthan I am updating the PC so seperated\nthe cases"
            # "FPGA and PI Data Rate 0.1\nPC Data Rate 0.33"
            # "_____________                           _"
            n59 = event-data() -> ()  [unwired: 1 in, 3 out]
            n60 = Unbundle By Name(w151) -> ("PC Data Timer"=w157:dbl, "PC Data Rate (sec)"=w144:dbl, "FPGA Data Timer"=w154:dbl, "FPGA Data Rate (sec)"=w153:dbl)
            n61 = Get Date/Time In Seconds() -> (seconds since 1Jan1904=w158:timestamp)
            n62 = To Double Precision Float(number=w158) -> (double precision float=w150:dbl)
            n63 = Subtract(x=w150, y=w157) -> (x-y=w156:dbl)
            n64 = Subtract(x=w150, y=w154) -> (x-y=w155:dbl)
            n65 = Greater?(x=w156, y=w144) -> (0:w152:bool)
            n66 = Greater?(x=w155, y=w153) -> (0:w148:bool)
            n67 = case shown="True" w152 {
              tunnel: [w170 w187] -> w149
              tunnel: w150 -> [_ w186]
              tunnel: w151 -> [w170 w175]
              tunnel: [FALSE "SaveConfig"] -> w145
              frame False {
              }
              frame True {
                # "For debug"
                n68 = Unbundle By Name(w175) -> ("AveDataCluster"=w177:T2)
                n69 = disable-structure shown="Disabled" {
                  frame Disabled {
                    n70 = call "Open or Closed Loop.vi"("Mode"=enum16{"Init", "Settings", "Run"}."Settings", "VDirect"="VDirect", "DirectV?"="DirectV?", "PresDirect"="PresDirect", "DirectPres?"="DirectPres?") -> ()  [unwired: 9 in, 2 out]
                  }
                  frame Enabled {
                  }
                }
                n71 = Flatten To String(anything=w177) -> (data string=w176:string)  [unwired: 3 in, 2 out]
                n72 = Bundle(cluster=T13 {"Command"="", "FlattenedData"=""}, "Command"="Data", "FlattenedData"=w176) -> (w179:T13)
                n73 = Flatten To String(anything=w179) -> (data string=w184:string)  [unwired: 3 in, 2 out]
                n74 = Bundle By Name(cluster=w175, "PC Data Timer"=w186, "CommandCluster"="CmdCluster", "PS Enable"="PS Enable", "ControlArray"="ControlArray", "DesiredCluster"="DesiredCluster") -> (w187:T12)
                n75 = call "RT Send Event.vi"("RTsend/PCrecv CMD"=RTsend_PCrecv_CMD."Data" ("RT Send Command"), "Mode"=Event_Mode."Set", "Flattened Data"=w184) -> ()  [unwired: 11 in, 2 out]
              }
            }
            n76 = case shown="True" w148 {
              tunnel: w143 -> [w165 w169]
              tunnel: [w165 w168] -> w147
              frame False {
              }
              frame True {
                n77 = Insert Into Array(array=w169, index=0, new element=string[] ["Read Data", "PI Controller"]) -> (w168:string[])
              }
            }
            n78 = case shown="True" w145 {
              tunnel: w147 -> [w160 w164]
              tunnel: [w160 w163] -> w146
              frame False {
              }
              frame True {
                n79 = Insert Into Array(array=w164, index=0, new element=string[] ["Save Config"]) -> (w163:string[])
              }
            }
          }
          event User Event {
            n80 = event-data() -> ("PCsend/RTrecv CMD"=w194:T16, "Flattened Data"=w198:string)  [unwired: 1 in]
            n81 = case shown="\"Controller\"" w194 {
              tunnel: w200 -> [w203 w205 w208 w216 w270 w286 w292 w305 w323 w331 w335 w341 w353]
              tunnel: [w203 w205 w208 w231 w282 w285 w292 w315 w323 w330 w334 w341 w352] -> w199
              tunnel: w198 -> [_ _ _ w232 w281 w288 _ w314 _ w329 w339 w347 w355]
              tunnel: w197 -> [w202 w204 w207 w233 w263 w284 w302 w304 w319 w326 w338 w346 w351]
              tunnel: [w202 w204 w207 w233 w262 w284 w302 w304 w319 w326 w338 w346 w351] -> w196
              tunnel: w193 -> [w201 w206 w209 w234 w277 w290 w303 w313 w322 w332 w337 w348 w354]
              tunnel: [w201 w206 w209 w234 w277 w289 w303 w313 w321 w332 w337 w348 w354] -> w195
              frame Default {
                # "Shouldn't ever get here\nwhich would mean something is not setup correctly"
              }
              frame "ConnSettings" {
              }
              frame "Connect" {
              }
              frame "CMD" {
                # "command\n\n___________\n\ndesired"
                # "This changes from visual view to correctly\nassigning the indirect parameters to the\ndirect control that most closely correlates"
                n82 = Unbundle By Name(w216) -> ("Tolerances"=w215:dbl[])
                n83 = Unflatten From String(type=T14 {"CommandCluster"={"Para1"=0, "SP1"=0.0, "Para2"=0, "SP2"=0.0, "Para3"=0, "SP3"=0.0}, "DesiredCluster"={"Para1"=0, "SP1"=0.0, "Para2"=0, "SP2"=0.0, "Para3"=0, "SP3"=0.0}}, binary string=w232) -> (value=w228:T14)  [unwired: 3 in, 2 out]
                n84 = Unbundle By Name(w228) -> ("CommandCluster.Para1"=w223:i32, "CommandCluster.SP1"=w226:dbl, "CommandCluster.Para2"=w224:i32, "CommandCluster.SP2"=w225:dbl, "DesiredCluster.Para1"=w210:i32, "DesiredCluster.SP1"=w211:dbl, "DesiredCluster.Para2"=w212:i32, "DesiredCluster.SP2"=w213:dbl)
                n85 = Equal To 0?(x=w223) -> (x = 0?=w227:bool)
                n86 = case shown="False" w227 {
                  tunnel: w228 -> [w244 w245]
                  tunnel: [w243 w245] -> w218
                  tunnel: w223 -> [w242 _]
                  tunnel: w226 -> [w241 _]
                  tunnel: w224 -> [w240 _]
                  tunnel: w225 -> [w239 _]
                  tunnel: w213 -> [w238 _]
                  tunnel: w212 -> [w237 _]
                  tunnel: w211 -> [w236 _]
                  tunnel: w210 -> [w235 _]
                  frame False {
                    # "switch"
                    n87 = Bundle By Name(cluster=w244, "CommandCluster.Para2"=w242, "CommandCluster.SP2"=w241, "CommandCluster.Para1"=w240, "CommandCluster.SP1"=w239, "DesiredCluster.Para2"=w235, "DesiredCluster.SP2"=w236, "DesiredCluster.Para1"=w237, "DesiredCluster.SP1"=w238) -> (w243:T14)
                  }
                  frame True {
                  }
                }
                n88 = Unbundle By Name(w218) -> ("CommandCluster.Para2"=w230:i32)
                n89 = Unbundle(w218) -> ("CommandCluster"=w219:T1, "DesiredCluster"=w217:T1)
                n90 = Equal?(x=w230, y=4) -> (x = y?=w222:bool)
                n91 = call "Create Tolerance Bands.vi"("DesiredCluster"=w217, "Tolerances"=w215) -> ("BoundsArray"=w214:dbl[][])  [unwired: 13 in]
                n92 = local write "DesiredCluster"(w217) -> ()
                n93 = local write "CmdCluster"(w219) -> ()
                n94 = Bundle By Name(cluster=w216, "CommandCluster"=w219, "DesiredCluster"=w217, "FreezeCmdPID"=FALSE, "Deadhead?"=w222, "TolBands"=w214) -> (w231:T12)
              }
              frame "Controller" {
                w280 = 0  # Controller Index
                # "Don't need to know PWM?\nbecause that is handled by\nonly CAN controllers having\na subVI in the bottom loop"
                n95 = Unbundle By Name(w270) -> ("Controller List"=w252:T5, "PS Enable"=w269:bool, "ControlArray"=w256:T3)
                n96 = Unflatten From String(type=w280, binary string=w281) -> (value=w279:i32)  [unwired: 3 in, 2 out]
                n97 = Index Array(array=w252, index=w279) -> (element=w278:T6)
                n98 = Unbundle By Name(w278) -> ("Controller Name"=→"Controller Name":T4, "CommSeg"=w258:i32, "Solenoid Stop?"=w267:bool, "Frequency"=w266:i32, "Stop Command"=w247:dbl, "Command Step"=w255:dbl, "High Command"=w254:dbl, "Low Command"=w253:dbl, "Indirect Nonzero CMD"=w251:dbl)
                n99 = call "Set Controller Limits.vi"("IndMin"=w251, "Min"=w253, "Max"=w254, "StepSize"=w255, "ControlArray In"=w256) -> ("ControlArray Out"=w250:T3)  [unwired: 10 in]
                n100 = Divide(x=40000000.0 ("PWM Period (Ticks)"), y=w266) -> (x/y=w272:dbl)
                n101 = Divide(x=w272, y=100.0 ("PWM Period (Ticks)")) -> (x/y=w259:dbl)
                n102 = To Unsigned Long Integer(number=w272) -> (unsigned 32bit integer=w274:u32)
                n103 = Equal?(x=w258, y=2) -> (x = y?=w257:bool)
                n104 = Select(t=FALSE, s=w267, f=w269) -> (s? t:f=w264:bool)
                n105 = Not(x=w257) -> (.not. x?=w248:bool)
                n106 = Insert Into Array(array=w263, index=0, new element=string[] ["Load Controller Settings", "Save Config"]) -> (w262:string[])
                n107 = Multiply(x=w259, y=w247) -> (x*y=w271:dbl)
                n108 = To Long Integer(number=w271) -> (32bit integer=w249:i32)
                n109 = Bundle By Name(cluster=w270, "CMD Scaler"=w259, "Controller"=w278, "PWM Period (ticks)"=w274, "ControlArray"=w250, "PS Enable"=w264) -> (w282:T12)
                n110 = local write "PS Enable"(w264) -> ()
                n111 = local write "ControlArray"(w250) -> ()
                n112 = local write "CommSegs"(w258) -> ()
                n113 = local write "Brushed Speed"(w248) -> ()
                n114 = xnode "Read/Write Control"("FPGA VI Reference In"=w277, "Brushed Speed"=FALSE, "PWM Period (ticks)"=w274, "PWM Duty"=w249) -> ()  [unwired: 1 in, 2 out]
              }
              frame "PSenable" {
                n115 = Unflatten From String(type=FALSE, binary string=w288) -> (value=w283:bool)  [unwired: 3 in, 2 out]
                n116 = Bundle By Name(cluster=w286, "PS Enable"=w283) -> (w285:T12)
                n117 = xnode "Read/Write Control"("FPGA VI Reference In"=w290, "PSenable"=w283) -> ("FPGA VI Reference Out"=w289:refnum<k20>)  [unwired: 1 in, 1 out]
                n118 = local write "PS Enable"(w283) -> ()
              }
              frame "ReqCalDate" {
                n119 = Unbundle By Name(w292) -> ("Version"=w291:u8)
                n120 = local read "PrevCalDate"() -> (w294:i32)
                n121 = Bundle("PrevCalDate"=w294, "Version"=w291) -> (w293:cluster{"PrevCalDate":i32, "Version":u8})  [unwired: 1 in]
                n122 = Flatten To String(anything=w293) -> (data string=w295:string)  [unwired: 3 in, 2 out]
                n123 = Bundle(cluster=T13 {"Command"="", "FlattenedData"=""}, "Command"="CalFileDate", "FlattenedData"=w295) -> (w297:T13)
                n124 = Flatten To String(anything=w297) -> (data string=w300:string)  [unwired: 3 in, 2 out]
                n125 = call "RT Send Event.vi"("RTsend/PCrecv CMD"=RTsend_PCrecv_CMD."CalFileDate" ("RT Send Command"), "Mode"=Event_Mode."Set", "Flattened Data"=w300) -> ()  [unwired: 11 in, 2 out]
              }
              frame "Tolerances" {
                w306 = T17 {"Voltage Tolerances"=0.0, "Pressure Tolerances"=0.0, "Flow Tolerances"=0.0, "Speed Tolerances"=0.0, "Stable Count (sec)"=0.0}  # Stability Cluster
                n126 = Unflatten From String(type=w306, binary string=w314) -> (value=w312:T17)  [unwired: 3 in, 2 out]
                n127 = Unbundle By Name(w312) -> ("Voltage Tolerances"=w311:dbl, "Pressure Tolerances"=w310:dbl, "Flow Tolerances"=w309:dbl, "Speed Tolerances"=w308:dbl)
                n128 = Build Array(w311, w310, w309, w308) -> (w307:dbl[])
                n129 = Bundle By Name(cluster=w305, "Tolerances"=w307) -> (w315:T12)
              }
              frame "Stable Trigger" {
                n130 = xnode "Read/Write Control"("FPGA VI Reference In"=w322, "StableTrigger"=fxp<+/-,20,5> 5.0) -> ("FPGA VI Reference Out"=w317:refnum<k20>)  [unwired: 1 in, 1 out]
                n131 = flat-sequence {
                  tunnel: w317 -> [w325]
                  tunnel: [w325] -> w316
                  frame #0 {
                    n132 = Wait (ms)(milliseconds to wait=u32 10) -> ()  [unwired: 1 out]
                  }
                }
                n133 = xnode "Read/Write Control"("FPGA VI Reference In"=w316, "StableTrigger"=fxp<+/-,20,5> 0.0) -> ("FPGA VI Reference Out"=w321:refnum<k20>)  [unwired: 1 in, 1 out]
              }
              frame "VPLimits" {
                n134 = Unflatten From String(type=dbl[] [], binary string=w329) -> (value=w327:dbl[])  [unwired: 3 in, 2 out]
                n135 = Bundle By Name(cluster=w331, "VandPLimit"=w327) -> (w330:T12)
              }
              frame "NeedleValve" {
                n136 = Unflatten From String(type=FALSE, binary string=w339) -> (value=w336:bool)  [unwired: 3 in, 2 out]
                n137 = Not(x=w336) -> (.not. x?=w333:bool)
                n138 = xnode "Read/Write Control"("FPGA VI Reference In"=w337, "NeedleValve"=w333) -> ()  [unwired: 1 in, 2 out]
                n139 = Bundle By Name(cluster=w335, "NeedleValve"=w333) -> (w334:T12)
              }
              frame "SpeedWindow" {
                n140 = Unflatten From String(type=cluster{u16, u16} {0, 0}, binary string=w347) -> (value=w345:cluster{u16, u16})  [unwired: 3 in, 2 out]
                n141 = Unbundle(w345) -> (w343:u16, w342:u16)
                n142 = local write "Min Window"(w343) -> ()
                n143 = local write "Max Window"(w342) -> ()
              }
              frame "FreezeCmdPID" {
                n144 = Unflatten From String(type=FALSE, binary string=w355) -> (value=w349:bool)  [unwired: 3 in, 2 out]
                n145 = Bundle By Name(cluster=w353, "FreezeCmdPID"=w349) -> (w352:T12)
              }
            }
          }
        }
      }
      frame "Read Data" {
        # "At a startup the first reading is saturation when controlling\nto speed with voltage that means the voltage is dropped to\ncompensate which then the pump just pulses on/off"
        # "Efficiency % = ( 36 * Pressure * Flow ) / ( Voltage * Current )"
        n146 = Get Date/Time In Seconds() -> (seconds since 1Jan1904=w357:timestamp)
        n147 = flat-sequence {
          tunnel: w359 -> [w395]
          tunnel: [w394] -> w358
          tunnel: w357 -> [w393]
          tunnel: w356 -> [w368]
          frame #0 {
            w367 = 10 ("ave pts")
            # "Do not need instant efficiency so only doing average\nefficiency to have one less averaging function"
            # "CommSeg is coming through as 2, 8, or 10"
            n148 = Unbundle By Name(w368) -> ("InstDataCluster"=w391:T2, "Cal Coeffs"=w378:dbl[][])
            n149 = xnode "Read/Write Control"("FPGA VI Reference In"=w395) -> ("DataCluster"=w375:T18)  [unwired: 1 in, 2 out]
            n150 = Cluster To Array(cluster=w375) -> (array=w373:fxp<+/-,25,15>[])
            n151 = local read "Speed"() -> (w372:dbl)
            n152 = To Double Precision Float(number=w373) -> (double precision float=w361:dbl[])
            n153 = Replace Array Subset(array=w361, new element=w372, index=7) -> (w379:dbl[])
            n154 = call "Calibration Applier.vi"("Cal Coefficients"=w378, "Data In"=w379) -> ("Data Cluster"=w377:T19)  [unwired: 13 in]
            n155 = call "AI RT FIFO.vi"("Data IN"=w379, "Mode"=Stream_RT_FIFO_Mode."Write") -> ()  [unwired: 11 in, 3 out]
            n156 = Unbundle(w377) -> ("[0]"=w385:dbl, "[1]"=w386:dbl, "[2]"=w376:dbl, "[3]"=w382:dbl, "[4]"=w381:dbl, "[5]"=w380:dbl, "[6]"=w384:dbl, "[7]"=w383:dbl)
            n157 = call <vilib>:"Mean PtByPt.vi"("x"=w386, "sample length"=w367) -> ("mean"=w388:dbl)  [unwired: 2 in, 1 out]
            n158 = call <vilib>:"Mean PtByPt.vi"("x"=w382, "sample length"=w367) -> ("mean"=w366:dbl)  [unwired: 2 in, 1 out]
            n159 = call <vilib>:"Mean PtByPt.vi"("x"=w380, "sample length"=w367) -> ("mean"=w365:dbl)  [unwired: 2 in, 1 out]
            n160 = call <vilib>:"Mean PtByPt.vi"("x"=w383, "sample length"=w367) -> ("mean"=w387:dbl)  [unwired: 2 in, 1 out]
            n161 = call <vilib>:"Mean PtByPt.vi"("x"=w385, "sample length"=w367) -> ("mean"=w389:dbl)  [unwired: 2 in, 1 out]
            n162 = call <vilib>:"Mean PtByPt.vi"("x"=w376, "sample length"=w367) -> ("mean"=w364:dbl)  [unwired: 2 in, 1 out]
            n163 = call <vilib>:"Mean PtByPt.vi"("x"=w381, "sample length"=w367) -> ("mean"=w363:dbl)  [unwired: 2 in, 1 out]
            n164 = call <vilib>:"Mean PtByPt.vi"("x"=w384, "sample length"=w367) -> ("mean"=w390:dbl)  [unwired: 2 in, 1 out]
            n165 = call "Efficiency Calculation.vi"("Current"=w365, "Voltage"=w363, "Flow"=w366, "Pressure"=w364) -> ("%Efficiency"=w362:dbl)  [unwired: 7 in]
            n166 = Bundle By Name(cluster=w391, "Pump Voltage (V)"=w385, "Pump Current (Arms)"=w386, "Pressure (kPA)"=w376, "Flow (L/H)"=w382, "Controller Voltage (V)"=w381, "Controller Current (A)"=w380, "Fuel Temp (C)"=w384, "Speed (RPM)"=w383) -> (w369:T2)
            n167 = Bundle By Name(cluster=w391, "Pump Voltage (V)"=w389, "Pump Current (Arms)"=w388, "Pressure (kPA)"=w364, "Flow (L/H)"=w366, "Controller Voltage (V)"=w363, "Controller Current (A)"=w365, "Fuel Temp (C)"=w390, "Speed (RPM)"=w387, "Efficiency (%)"=w362) -> (w370:T2)
            "Ave Data Cluster" <- w370
            n168 = To Double Precision Float(number=w393) -> (double precision float=w392:dbl)
            n169 = Bundle By Name(cluster=w368, "FPGA Data Timer"=w392, "InstDataCluster"=w369, "AveDataCluster"=w370) -> (w394:T12)
          }
        }
      }
      frame "PI Controller" {
        w424 = fxp<+/-,20,5> 0.0 ("VoltCtrl")
        n170 = Unbundle By Name(w429) -> ("AveDataCluster"=w396:T2, "InstDataCluster"=w397:T2, "ControlArray"=w400:T3, "Controller.Stop Command"=w407:dbl, "NeedleValve"=w406:bool, "CommandCluster"=w403:T1, "VandPLimit"=w402:dbl[], "Controller.Controller?"=w401:bool, "FreezeCmdPID"=w404:bool, "Controller.PWM?"=w413:bool, "Deadhead?"=w414:bool, "PS Enable"=w416:bool, "CMD Scaler"=w415:dbl, "TolBands"=w398:dbl[][])
        n171 = call "Data Cluster to Feedback Array.vi"("InstDataCluster"=w397) -> ("Inst FB"=w405:dbl[])  [unwired: 2 in]
        n172 = call "PID for Voltage.vi"("ControlArray"=w400, "Feedback"=w405, "CommandCluster"=w403, "VandPLimits"=w402, "Controller?"=w401) -> ("PIdata"=w411:dbl[], "Output"=w421:dbl)  [unwired: 9 in]
        n173 = Not(x=w414) -> (.not. x?=w408:bool)
        n174 = call "PID for Pressure.vi"("ControlArray"=w400, "NeedleValve"=w406, "Feedback"=w405, "CommandCluster"=w403, "VandPLimits"=w402, "Run?"=w408, "Controller?"=w401) -> ("PIdata"=w410:dbl[], "Output"=w420:dbl)  [unwired: 7 in]
        n175 = call "PID for Controller Command.vi"("ControlArray"=w400, "Stop CMD"=w407, "Feedback"=w405, "CommandCluster"=w403, "FreezeCmdPID"=w404, "Run?"=w401, "Controller?"=w401) -> ("PIdata"=w409:dbl[], "Output"=w412:dbl)  [unwired: 6 in, 1 out]
        n176 = call "Open or Closed Loop.vi"("VPID"=w421, "PresPID"=w420) -> ("VSig"=w419:dbl, "PresSig"=w417:dbl)  [unwired: 12 in]
        n177 = local read "GraphTab"() -> (w418:enum32{"Page 1", "Page 2"})
        n178 = call "Graph Prep.vi"("V_PIdata"=w411, "InstDataCluster"=w397, "AveDataCluster"=w396, "Enable Graphs"="Enable Graphs", "GraphTab"=w418, "Pres_PIdata"=w410, "CMD_PIdata"=w409, "VSig"=w419, "PresSig"=w417, "CMDSig"=w412, "Controller?"=w401, "TolBounds"=w398, "CommandCluster"=w403) -> ()  [unwired: 3 in]
        n179 = disable-structure shown="Enabled" {
          disable-tunnel: w427 -> [w431 w437]
          disable-tunnel: [w430 w437] -> w426
          frame Disabled {
            # "Deadhead or Controller CMD (ie 4) will skip PID"
            n180 = case shown="True" {
              selector: _ -> [_ _]
              tunnel: w431 -> [w432 w436]
              tunnel: [w432 w435] -> w430
              frame False {
              }
              frame True {
                n181 = Insert Into Array(array=w436, index=0, new element="Stable Trigger" ("new element/subarray")) -> (w435:string[])
              }
            }
          }
          frame Enabled {
            # "Now calculating stable on PC\nto determine when to send stable trigger\nfor NVH purposes would need to send\nTCP message that triggers it"
          }
        }
        n182 = To Fixed-Point(fixed-point type=w424, number=w419) -> (fixed-point=w422:fxp<+/-,20,5>)
        n183 = To Fixed-Point(fixed-point type=w424, number=w417) -> (fixed-point=w423:fxp<+/-,20,5>)
        n184 = Bundle By Name(cluster=w429, "AveDataCluster.Controller CMD"=w412, "InstDataCluster.Controller CMD"=w412) -> (w425:T12)
        n185 = case shown="True" w413 {
          tunnel: w428 -> [w441 w453]
          tunnel: w414 -> [w442 w452]
          tunnel: w422 -> [w443 w451]
          tunnel: w423 -> [w444 w450]
          tunnel: w416 -> [w439 w449]
          tunnel: w412 -> [w438 w446]
          tunnel: w415 -> [_ w445]
          frame False {
            n186 = To Unsigned Word Integer(number=w438) -> (unsigned 16bit integer=w440:u16)
            n187 = xnode "Read/Write Control"("FPGA VI Reference In"=w441, "Deadhead"=w442, "VoltCtrl"=w443, "PresCtrl"=w444, "PSenable"=w439) -> ()  [unwired: 1 in, 2 out]
            n188 = local write "CAN CMD"(w440) -> ()
          }
          frame True {
            n189 = Multiply(x=w445, y=w446) -> (x*y=w447:dbl)
            n190 = To Long Integer(number=w447) -> (32bit integer=w448:i32)
            n191 = xnode "Read/Write Control"("FPGA VI Reference In"=w453, "Deadhead"=w452, "VoltCtrl"=w451, "PresCtrl"=w450, "PSenable"=w449, "PWM Duty"=w448) -> ()  [unwired: 1 in, 2 out]
          }
        }
      }
      frame "Stable Trigger" {
        n192 = Unbundle By Name(w458) -> ("InstDataCluster.Stabilized?"=w457:bool)
        n193 = Select(t=fxp<+/-,20,5> 5.0 ("StableTrigger"), s=w457, f=fxp<+/-,20,5> 0.0 ("StableTrigger")) -> (s? t:f=w456:fxp<+/-,20,5>)
        n194 = xnode "Read/Write Control"("FPGA VI Reference In"=w460, "StableTrigger"=w456) -> ("FPGA VI Reference Out"=w459:refnum<k20>)  [unwired: 1 in, 1 out]
      }
      frame "Load Controller Settings" {
        n195 = Unbundle By Name(w467) -> ("Controller.Name"=w465:string, "ControlArray"=w471:T3)
        n196 = Unbundle By Name(w467) -> ("Controller.Command Step"=w470:dbl, "Controller.High Command"=w469:dbl, "Controller.Low Command"=w468:dbl, "Controller.Indirect Nonzero CMD"=w464:dbl)
        n197 = call "RW Controller Settings.vi"("Filepath"=path "c:/Controller Settings.ini", "Read (F)"=TRUE, "Controller Name"=w465, "ControlArray In"=w471) -> ("ControlArray Out"=w466:T3)  [unwired: 10 in, 1 out]
        n198 = call "Set Controller Limits.vi"("IndMin"=w464, "Min"=w468, "Max"=w469, "StepSize"=w470, "ControlArray In"=w466) -> ("ControlArray Out"=w463:T3)  [unwired: 10 in]
        n199 = local write "ControlArray"(w463) -> ()
        n200 = Bundle By Name(cluster=w467, "ControlArray"=w463) -> (w473:T12)
      }
      frame "Save Config" {
        n201 = local read "ControlArray"() -> (w477:T3)
        n202 = Unbundle By Name(w479) -> ("Controller.Name"=w480:string)
        n203 = call "RW Controls INI.vi"("Filepath"=path "c:/Controls.ini", "ControlArray In"=w477) -> ("ControlArray Out"=w476:T3, "Error Out"=w485:errorcluster)  [unwired: 12 in]
        n204 = call <vilib>:"Clear Errors.vi"("error in (no error)"=w485) -> ("error out"=w484:errorcluster)  [unwired: 6 in]
        n205 = call "RW Controller Settings.vi"("Filepath"=path "c:/Controller Settings.ini", "Controller Name"=w480, "ControlArray In"=w476, "Error In"=w484) -> ("ControlArray Out"=w482:T3, "Error Out"=w483:errorcluster)  [unwired: 10 in]
        n206 = call <vilib>:"Clear Errors.vi"("error in (no error)"=w483) -> ()  [unwired: 6 in, 1 out]
        n207 = Bundle By Name(cluster=w479, "ControlArray"=w482) -> (w486:T12)
      }
    }
  }
  n208 = call "CAN Communication.vi"("CAN Mode"=CAN_Mode."Init", "Error IN"=w7) -> ("Error OUT"=w23:errorcluster)  [unwired: 8 in, 1 out]
  n209 = call "RT Engine.vi"("Error In"=w7) -> ()  [unwired: 11 in]
  n210 = flat-sequence {
    tunnel: w19 -> [w489]
    frame #0 {
      n211 = Wait on Occurrence(2:w489) -> ()  [unwired: 2 in, 1 out]
    }
    frame #1 {
      n212 = call "AI RT FIFO.vi"("Mode"=Stream_RT_FIFO_Mode."Create", "Buffer Size"=800, "# of elements"=8) -> ()  [unwired: 10 in, 3 out]
    }
    frame #2 {
      n213 = control-ref of="Stream Stop"() -> (w495:refnum<vi>)
      n214 = property class="Bool (strict)"(reference=w495, "Value"=FALSE) -> (reference out=w493:refnum<vi>)  [unwired: 1 in, 1 out]
      n215 = call "Loop (Data Stream).vi"("Stop"=w493) -> ()  [unwired: 10 in, 1 out]
    }
    frame #3 {
      n216 = call "AI RT FIFO.vi"("Mode"=Stream_RT_FIFO_Mode."Delete") -> ()  [unwired: 12 in, 3 out]
    }
  }
  n217 = while {
    tunnel: w9 -> [w511]
    shift-right: [w505] -> _
    shift-left: _ -> [w504]
    stop <- FALSE stop-if-true
    n218 = xnode "Read/Write Control"("FPGA VI Reference In"=w511) -> ("FPGA VI Reference Out"=w510:refnum<k20>, "Actual Loop Time"=→"Actual Loop Time":u32, "Actual Loop Time 2"=→"Actual Loop Time 2":u32)  [unwired: 1 in, 1 out]
    n219 = xnode "Invoke Method"("FPGA VI Reference In"=w510, "Number of Elements"=u32 0) -> ("FPGA VI Reference Out"=w513:refnum<k20>, "Elements Remaining"=w514:u32)  [unwired: 2 in, 2 out]
    n220 = Wait (ms)(milliseconds to wait=u32 100) -> ()  [unwired: 1 out]
    n221 = Get Date/Time In Seconds() -> (seconds since 1Jan1904=w507:timestamp)
    n222 = To Double Precision Float(number=w507) -> (double precision float=w505:dbl)
    n223 = xnode "Invoke Method"("FPGA VI Reference In"=w513, "Number of Elements"=w514) -> ("Data"=w503:fxp<+/-,24,5>[])  [unwired: 2 in, 3 out]
    n224 = Subtract(x=w505, y=w504) -> (x-y=→"Speed Loop Time":dbl)
    n225 = To Double Precision Float(number=w503) -> (double precision float=w501:dbl[])
    n226 = case shown="True" "Brushed Speed" {
      tunnel: w501 -> [w522 w524]
      tunnel: [w519 w523] -> w502
      tunnel: "CommSegs" -> [w518 _]
      tunnel: "Min Window" -> [w521 _]
      tunnel: "Max Window" -> [w520 _]
      frame True {
        n227 = To Double Precision Float(number=w518) -> (double precision float=w517:dbl)
        n228 = call "GetSpeed.vi"("Max Window"=w520, "Min Window"=w521, "Y"=w522, "comm seg"=w517) -> ("Speed"=w519:dbl)  [unwired: 6 in, 1 out]
      }
      frame False {
        n229 = call "Brushless Speed Calc (RT).vi"("Data In"=w524) -> ("Speed"=w523:dbl)  [unwired: 14 in]
      }
    }
    "Speed" <- w502
  }
  n230 = while {
    tunnel: w23 -> [w531]
    i -> [w530]
    stop <- FALSE stop-if-true
    n231 = local read "Controller Name"() -> (w532:T4)
    n232 = Quotient & Remainder(x=w530, y=10) -> (x-y*floor(x/y)=w528:i32)  [unwired: 1 out]
    n233 = Equal To 0?(x=w528) -> (x = 0?=w527:bool)
    n234 = case shown="\"Hella E4LMF\"..\"Hella E4DCG 30mm\"" w532 {
      tunnel: w531 -> [_ w535 w538 w541 w543 w545]
      tunnel: w527 -> [_ _ w537 _ _ _]
      tunnel: "CAN CMD" -> [_ w534 w536 w540 w542 w544]
      frame Default {
        n235 = Wait (ms)(milliseconds to wait=u32 500) -> ()  [unwired: 1 out]
      }
      frame "Conti" {
        n236 = call "Conti CAN.vi"("Error IN"=w535, "CMD"=w534) -> ()  [unwired: 9 in, 1 out]
      }
      frame "Helbako (old)" {
        n237 = call "Helbako CAN.vi"("Split-timer"=w537, "Error IN"=w538, "CMD"=w536) -> ()  [unwired: 8 in, 1 out]
      }
      frame "Hella E4LMF".."Hella E4DCG 30mm" {
        n238 = To Unsigned Byte Integer(number=w540) -> (unsigned 8bit integer=w539:u8)
        n239 = call "Hella BLDC CAN.vi"("Error IN"=w541, "CMD"=w539) -> ()  [unwired: 9 in, 1 out]
      }
      frame "Hella Hyundai Gas" {
        n240 = call "Hella CAN Gas.vi"("Pressure Command (kPa)"=w542, "Error In"=w543) -> ()  [unwired: 12 in, 2 out]
      }
      frame "Hella Hyundai Diesel" {
        n241 = call "Hella CAN Diesel.vi"("Command (kPa)"=w544, "Error In"=w545) -> ()  [unwired: 13 in, 1 out]
      }
    }
  }
  n242 = while {
    tunnel: w7 -> [w548]
    stop <- FALSE stop-if-true
    n243 = call <vilib>:"RT Get CPU Loads.vi"("error in (no error)"=w548) -> ("CPU loads"=w551:T20[])  [unwired: 9 in, 1 out]
    n244 = Index Array(array=w551) -> (element=w550:T20)  [unwired: 1 in]
    n245 = Unbundle By Name(w550) -> ("Total (%)"=→"Total (%)":dbl)
    n246 = Wait (ms)(milliseconds to wait=u32 500) -> ()  [unwired: 1 out]
  }
